vi "photo Conversion.vi"(0 "KNR in":T1, 1 "順序":i32, 5 "error in":errorcluster, 6 "x1":i32, 7 "t1":i32, 8 "x2":i32, 9 "t2":i32, 10 "x3":i32, 11 "t3":i32) -> (12 "x":dbl, 14 "KNR out":T1, 19 "error out":errorcluster)   [LabVIEW 2013]
uses:
  <userlib>/KNR OS 3.0 LabVIEW Toolkit/Type Definition/KNR3 Reference.ctl
  <userlib>/_FPGA Interface Advanced Tools/FPGA Interface Base/FPGA Interface Base.lvclass
  <userlib>/KNR OS 3.0 LabVIEW Toolkit/Type Definition/Resource.ctl
panel:
  out "x33":i32
  out "x22":i32
  out "x11":i32
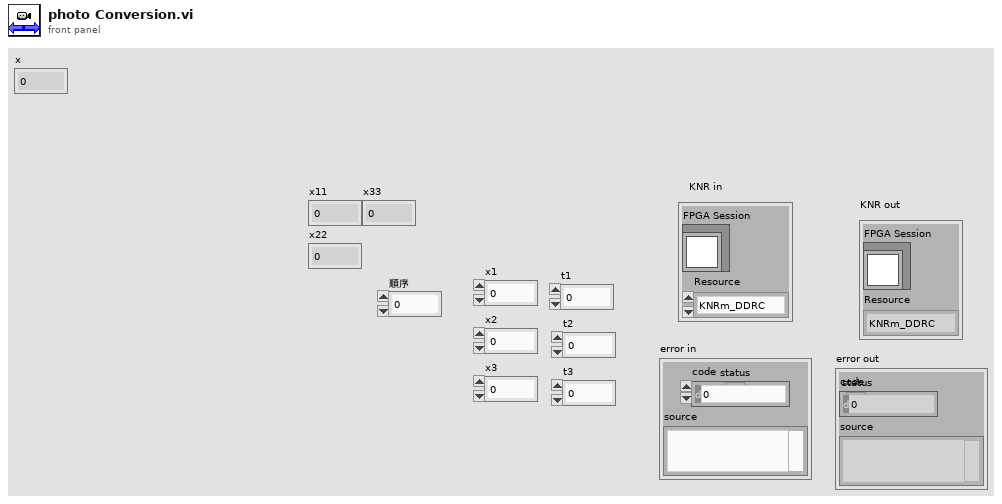
[diagram p1: front panel]
types:
  T1 = typedef "KNR3 Reference.ctl" = cluster{"FPGA Session":refnum<class "FPGA Interface Base.lvclass">, "Resource":T2}
  T2 = typedef "Resource.ctl" = enum16{"KNRm_DDRC", "KNRm_DDDD", "KNRm_DDDR", "KNRm_DDDC", "KNR"}
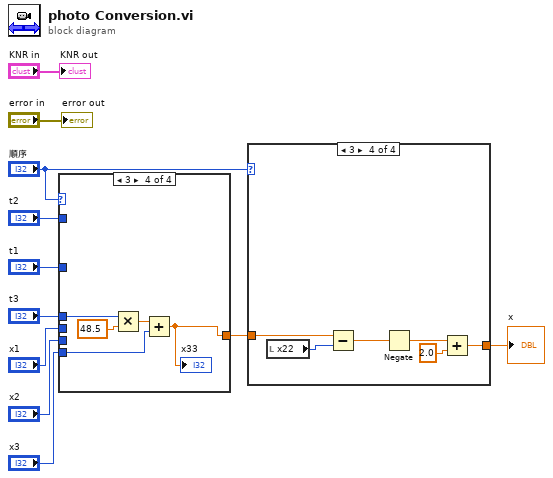
[diagram p0: block diagram]
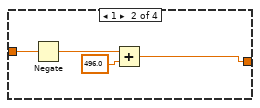
[diagram p3: hidden frame]
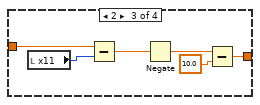
[diagram p4: hidden frame]
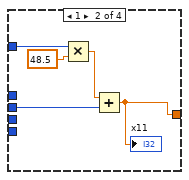
[diagram p6: hidden frame]
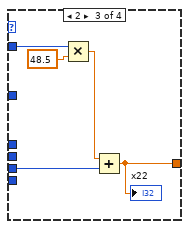
[diagram p7: hidden frame]
diagram:
  n1 = case shown="3" "順序" {
    tunnel: "t1" -> [_ w16 _ _]
    tunnel: "x1" -> [_ w14 _ _]
    tunnel: "t2" -> [_ _ w20 _]
    tunnel: "x2" -> [_ _ w19 _]
    tunnel: "t3" -> [_ _ _ w25]
    tunnel: "x3" -> [_ _ _ w24]
    tunnel: [_ w13 w18 w23] -> w5
    frame 0, Default {
    }
    frame 1 {
      n2 = Multiply(x=w16, y=48.5) -> (x*y=w15:dbl)
      n3 = Add(x=w15, y=w14) -> (x+y=w13:dbl)
      "x11" <- w13
    }
    frame 2 {
      n4 = Multiply(x=w20, y=48.5) -> (x*y=w21:dbl)
      n5 = Add(x=w21, y=w19) -> (x+y=w18:dbl)
      "x22" <- w18
    }
    frame 3 {
      n6 = Multiply(x=w25, y=48.5) -> (x*y=w26:dbl)
      n7 = Add(x=w26, y=w24) -> (x+y=w23:dbl)
      "x33" <- w23
    }
  }
  n8 = case shown="3" "順序" {
    tunnel: w5 -> [_ w30 w35 w42]
    tunnel: [_ w27 w31 w37] -> w1
    frame 0, Default {
    }
    frame 1 {
      n9 = Negate(x=w30) -> (-x=w28:dbl)
      n10 = Add(x=w28, y=496.0) -> (x+y=w27:dbl)
    }
    frame 2 {
      n11 = local read "x11"() -> (w36:i32)
      n12 = Subtract(x=w35, y=w36) -> (x-y=w34:dbl)
      n13 = Negate(x=w34) -> (-x=w33:dbl)
      n14 = Subtract(x=w33, y=10.0) -> (x-y=w31:dbl)
    }
    frame 3 {
      n15 = local read "x22"() -> (w41:i32)
      n16 = Subtract(x=w42, y=w41) -> (x-y=w40:dbl)
      n17 = Negate(x=w40) -> (-x=w39:dbl)
      n18 = Add(x=w39, y=2.0) -> (x+y=w37:dbl)
    }
  }
  "x" <- w1
  "KNR out" <- "KNR in"
  "error out" <- "error in"
